vi "Create or open log.vi"(8 "error in (no error)":errorcluster, 9 "Log string":string, 10 "Spreadsheet header string":string, 11 "appended path":path) -> (0 "error out":errorcluster, 3 "path":path)   [LabVIEW 2015]
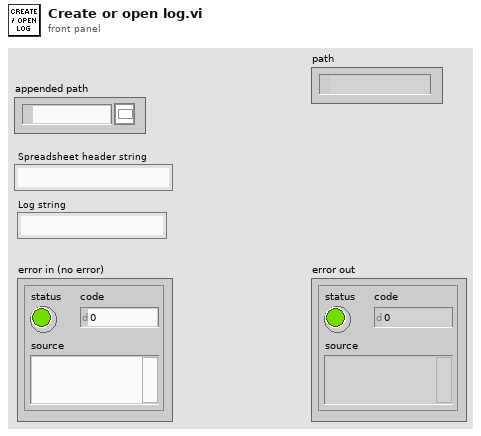
[diagram p1: front panel]
types:
  T1 = enum16{"open", "replace", "create", "open or create", "replace or create", "replace or create with confirmation"}
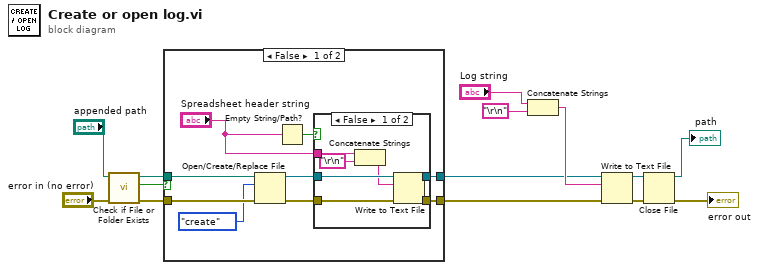
[diagram p0: block diagram]
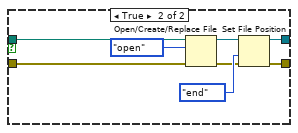
[diagram p3: hidden frame]
diagram:
  n1 = call <vilib>:"Check if File or Folder Exists.vi"("error in (no error)"="error in (no error)", "path"="appended path") -> ("error out"=w14:errorcluster, "file or folder exists?"=w11:bool, "dup path"=w12:path)  [unwired: 7 in]
  n2 = case shown="False" w11 {
    tunnel: w14 -> [w23 w40]
    tunnel: w12 -> [w21 w39]
    tunnel: [w18 w34] -> w3
    tunnel: [w17 w35] -> w4
    frame False {
      n3 = Open/Create/Replace File(file path (use dialog)=w21, error in=w23, operation (0:open)=T1."create") -> (refnum out=w19:refnum<file>, error out=w20:errorcluster)  [unwired: 3 in, 1 out]
      n4 = Empty String/Path?(string/path="Spreadsheet header string") -> (empty?=w16:bool)
      n5 = case shown="False" w16 {
        tunnel: w20 -> [w30 w31]
        tunnel: w19 -> [w29 w32]
        tunnel: [w28 w32] -> w18
        tunnel: [w27 w31] -> w17
        tunnel: "Spreadsheet header string" -> [w25 _]
        frame False {
          n6 = Concatenate Strings(w25, "\r\n") -> (w26:string)
          n7 = Write to Text File(file (use dialog)=w29, text=w26, error in=w30) -> (refnum out=w28:refnum<file>, error out=w27:errorcluster)  [unwired: 1 in, 1 out]
        }
        frame True {
        }
      }
    }
    frame True {
      n8 = Open/Create/Replace File(file path (use dialog)=w39, error in=w40, operation (0:open)=T1."open") -> (refnum out=w36:refnum<file>, error out=w37:errorcluster)  [unwired: 3 in, 1 out]
      n9 = Set File Position(refnum=w36, from (0:start)=enum16{"start", "end", "current"}."end", error in=w37) -> (refnum out=w34:refnum<file>, error out=w35:errorcluster)  [unwired: 1 in]
    }
  }
  n10 = Concatenate Strings("Log string", "\r\n") -> (w8:string)
  n11 = Write to Text File(file (use dialog)=w3, text=w8, error in=w4) -> (refnum out=w9:refnum<file>, error out=w7:errorcluster)  [unwired: 1 in, 1 out]
  n12 = Close File(refnum=w9, error in=w7) -> (path=→"path":path, error out=→"error out":errorcluster)
